vi "OpenAngleCriteria.vi"(8 "error in (no error)":errorcluster, 10 "point":dbl[](array[numeric]), 11 "PassObjective in":refnum<class "PassObjective.lvclass">) -> (0 "error out":errorcluster, 2 "evaluation":dbl, 3 "PassObjective out":refnum<class "PassObjective.lvclass">)   [LabVIEW 2023, in "PassObjective.lvclass"]
uses:
  PassObjective.lvclass
  PassObjective.lvclass/PassObjective.ctl
  Game_class/Game.lvclass/Game.ctl
  <vilib>/Analysis/_algsub.llb/Real Vector Norm.vi
  <vilib>/Analysis/baseanly.llb/Real Dot Product.vi
  Game_class/Read FieldRef.vi
  Field_class/Field.lvclass
  Utilities_class/Utilities.lvclass
  <vilib>/Analysis/NI_AALBase.lvlib
  <vilib>/Analysis/NI_AALPro.lvlib
  Game_class/Game.lvclass
panel:
  in  "minEval":dbl
  in  "maxAngle":dbl
  in  "minAngle":dbl
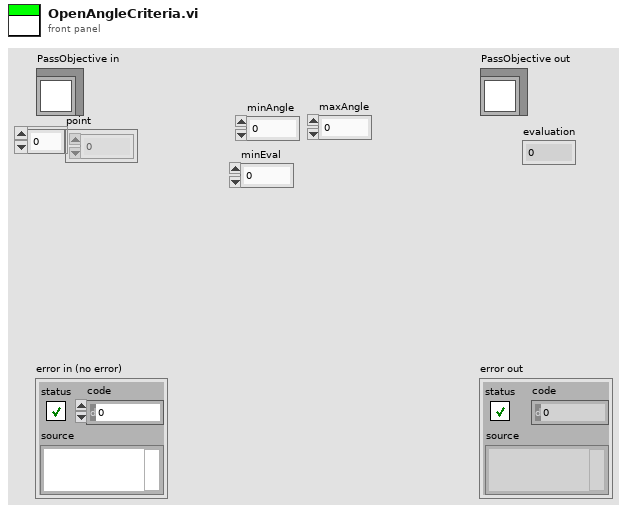
[diagram p1: front panel]
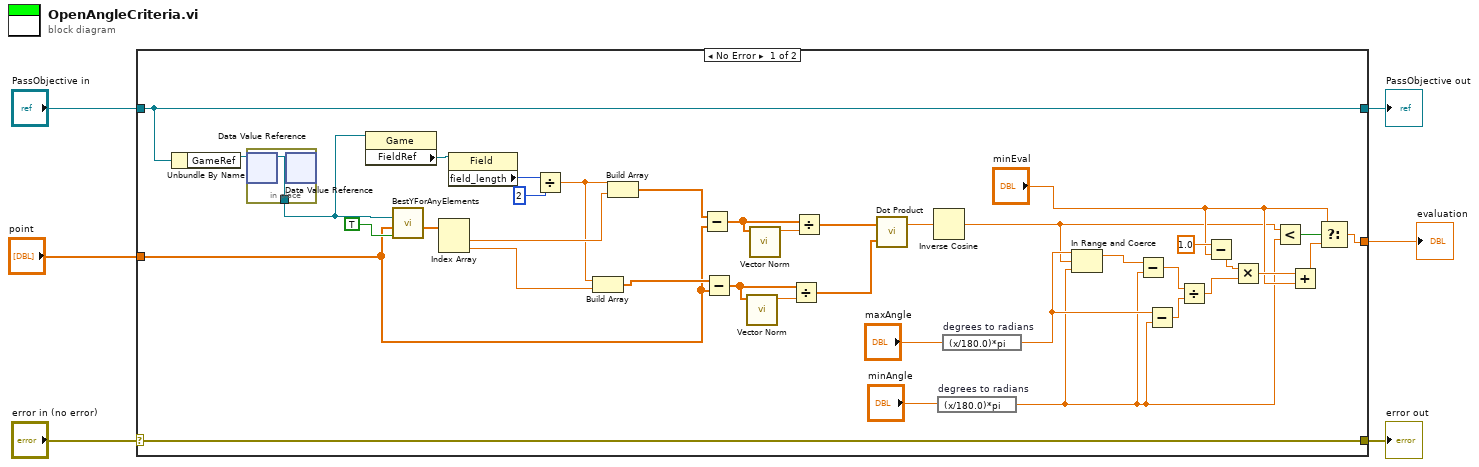
[diagram p0: block diagram]
diagram:
  n1 = case shown="No Error" "error in (no error)" {
    selector: "error in (no error)" -> [w44 w47]
    tunnel: [w44 w47] -> w5
    tunnel: [w42 w46] -> w3
    tunnel: "PassObjective in" -> [w42 w46]
    tunnel: "point" -> [w30 _]
    tunnel: [w25 _] -> w1
    frame No Error {
      n2 = Unbundle By Name(w42) -> ("GameRef"=w41:refnum<data-value>)
      n3 = in-place {
        in-place-border: [w45] -> w37
        n4 = in-place-dvr #1(w41) -> (w45:refnum<class "Game.lvclass">)  [unwired: 1 out]
        n5 = in-place-dvr #1() -> ()  [unwired: 1 in, 2 out]
      }
      n6 = property class="Game"(reference=w37) -> ("FieldRef"=w36:refnum<class "Field.lvclass">)  [unwired: 1 in, 2 out]
      n7 = call "BestYForAnyElements.vi"("inimigos"=TRUE, "Position to be analyzed"=w30, "Game"=w37) -> ("Gap Coord"=w40:dbl[])  [unwired: 5 in, 3 out]
      n8 = Index Array(array=w40) -> (element #1=w39:dbl, element #2=w38:dbl)  [unwired: 2 in]
      n9 = property class="Field"(reference=w36) -> ("field_length"=w35:i32)  [unwired: 1 in, 2 out]
      n10 = Divide(x=w35, y=2) -> (x/y=w33:dbl)
      n11 = Build Array(w33, w38) -> (w31:dbl[])
      n12 = Build Array(w33, w39) -> (w32:dbl[])
      n13 = Subtract(x=w32, y=w30) -> (x-y=w24:dbl[])
      n14 = Subtract(x=w31, y=w30) -> (x-y=w21:dbl[])
      n15 = call-poly <vilib>:"Vector Norm.vi"("Input Vector"=w21) -> ("norm"=w22:dbl)  [unwired: 9 in, 1 out]
      n16 = call-poly <vilib>:"Vector Norm.vi"("Input Vector"=w24) -> ("norm"=w23:dbl)  [unwired: 9 in, 1 out]
      n17 = Divide(x=w21, y=w22) -> (x/y=w19:dbl[])
      n18 = Divide(x=w24, y=w23) -> (x/y=w20:dbl[])
      n19 = call-poly <vilib>:"Dot Product.vi"("Y Vector"=w19, "X Vector"=w20) -> ("X * Y"=w29:dbl)  [unwired: 1 out]
      n20 = Inverse Cosine(1:w29) -> (0:w9:dbl)
      n21 = expression code="(x/180.0)*pi" "degrees to radians"("minAngle") -> (w8:dbl)
      n22 = expression code="(x/180.0)*pi" "degrees to radians"("maxAngle") -> (w10:dbl)
      n23 = In Range and Coerce(upper limit=w10, x=w9, lower limit=w8) -> (coerced(x)=w7:dbl)  [unwired: 1 out]
      n24 = Subtract(x=w7, y=w8) -> (x-y=w18:dbl)
      n25 = Subtract(x=w10, y=w8) -> (x-y=w17:dbl)
      n26 = Divide(x=w18, y=w17) -> (x/y=w16:dbl)
      n27 = Subtract(x=1.0, y="minEval") -> (x-y=w14:dbl)
      n28 = Multiply(x=w14, y=w16) -> (x*y=w13:dbl)
      n29 = Less?(x=w9, y=w8) -> (x < y?=w26:bool)
      n30 = Add(x=w13, y="minEval") -> (x+y=w12:dbl)
      n31 = Select(t="minEval", s=w26, f=w12) -> (s? t:f=w25:dbl)
    }
    frame Error {
    }
  }
  "error out" <- w5
  "PassObjective out" <- w3
  "evaluation" <- w1
